vi "gen_drive_waveform.vi"(11 "no of cycles":dbl=6000.0) -> (0 "signal out":waveform(dbl))   [LabVIEW 2019]
uses:
  global_variables.vi
  <vilib>/measure/NI_MABase.lvlib
panel:
  out "sample rate (from global)":dbl=500000.0 format="%#_6p"
  out "Transmit amplitude (from global)":dbl=3.3
  out "Transmit frequency (from global)":dbl=25000.0 format="%#_6p"
  out "Sample points per cycle":dbl
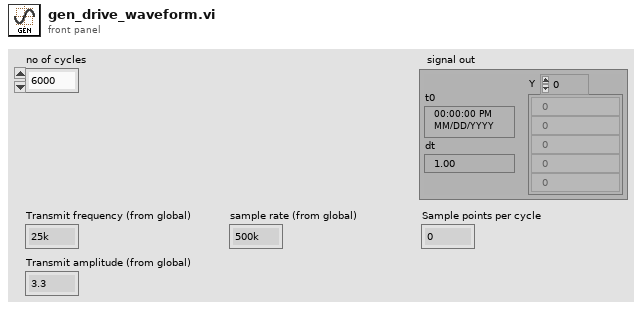
[diagram p1: front panel]
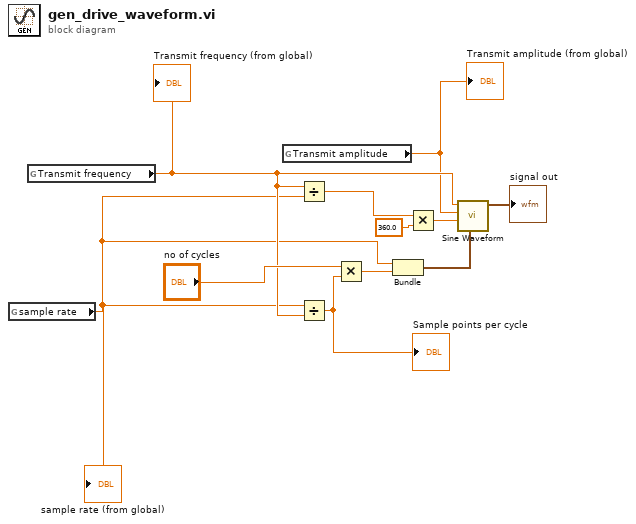
[diagram p0: block diagram]
diagram:
  n1 = global read "global_variables.vi" "sample rate"() -> (w2:dbl)
  "sample rate (from global)" <- w2
  n2 = global read "global_variables.vi" "Transmit frequency"() -> (w3:dbl)
  "Transmit frequency (from global)" <- w3
  n3 = global read "global_variables.vi" "Transmit amplitude"() -> (w1:dbl)
  "Transmit amplitude (from global)" <- w1
  n4 = Divide(x=w3, y=w2) -> (x/y=w10:dbl)
  n5 = Divide(x=w2, y=w3) -> (x/y=w5:dbl)
  "Sample points per cycle" <- w5
  n6 = Multiply(x="no of cycles", y=w5) -> (x*y=w4:dbl)
  n7 = Bundle("sample rate"=w2, w4) -> (w11:cluster{"sample rate":dbl, dbl})  [unwired: 1 in]
  n8 = Multiply(x=w10, y=360.0) -> (x*y=w8:dbl)
  n9 = call <vilib>:"Sine Waveform.vi"("sampling info"=w11, "phase"=w8, "amplitude"=w1, "frequency"=w3) -> ("signal out"=→"signal out":waveform(dbl))  [unwired: 6 in, 1 out]
